vi "Shutdown - Close Duplex.vi"(8 "error in (no error)":errorcluster, 11 "Duplex Packets":refnum<data-value>) -> (0 "error out":errorcluster)   [LabVIEW 2019, in "UDP-Custom-Device Engine.lvlib"]
uses:
  UDP-Custom-Device Engine.lvlib
  Shared/Types/Shared - Duplex Settings.ctl
  Shared/UDP-Custom-Device Shared.lvlib
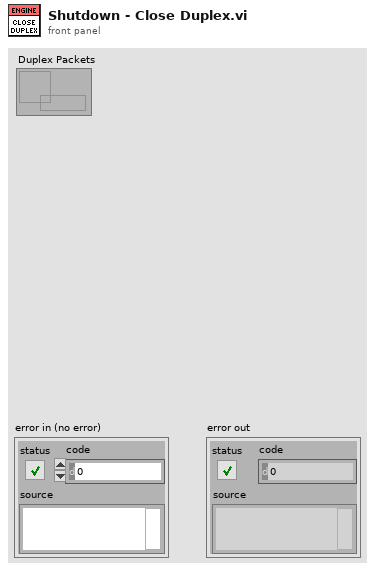
[diagram p1: front panel]
types:
  T1 = typedef "UDP-Custom-Device Shared.lvlib/Shared - Duplex Settings.ctl" = cluster{"Transmit Packet ID":i32, "Receive Packet ID":i32, "Multicast":bool, "Multicast Address":string, "IP Address":string, "Port":u16, "TTL":u16, "Duplex Connection":refnum<k16>}
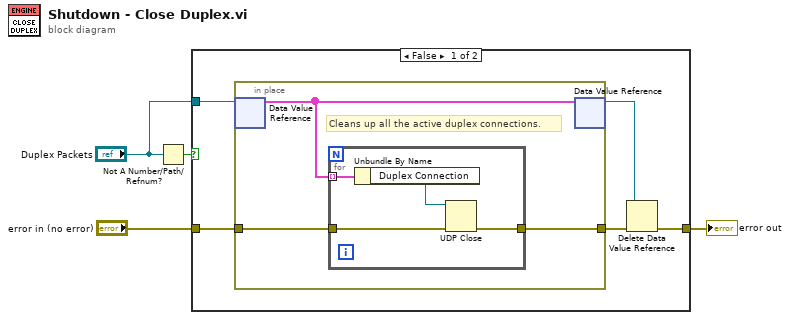
[diagram p0: block diagram]
diagram:
  n1 = Not A Number/Path/Refnum?(number/path/refnum="Duplex Packets") -> (NaN/Path/Refnum?=w2:bool)
  n2 = case shown="False" w2 {
    tunnel: "error in (no error)" -> [w9 w17]
    tunnel: [w6 w17] -> w3
    tunnel: "Duplex Packets" -> [w8 _]
    frame False {
      n3 = in-place {
        in-place-border: w9 -> [w12]
        in-place-border: [w11] -> w5
        # "Cleans up all the active duplex connections."
        n4 = in-place-dvr #1(w8) -> (w10:T1[])  [unwired: 1 out]
        n5 = for {
          tunnel: w10 -> [w16] mode=indexing
          tunnel: w12 -> [w14]
          tunnel: [w13] -> w11
          n6 = Unbundle By Name(w16) -> ("Duplex Connection"=w15:refnum<k16>)
          n7 = UDP Close(connection ID=w15, 8:w14) -> (error out=w13:errorcluster)  [unwired: 1 out]
        }
        n8 = in-place-dvr #1(w10) -> (w7:refnum<data-value>)  [unwired: 1 out]
      }
      n9 = Delete Data Value Reference(data value reference=w7, error in=w5) -> (error out=w6:errorcluster)  [unwired: 1 out]
    }
    frame True {
    }
  }
  "error out" <- w3
